vi "AutofocusContinuous.vi"() -> ()   [LabVIEW 2019]
uses:
  <vilib>/userDefined/High Color/IMAQdx.ctl
  include/GlobalVariables.vi
  Other Models/2010/Motion/AbortSingle.vi
  <vilib>/vision/NI_Vision_Development_Module.lvlib
  <vilib>/vision/driver/NI_Vision_Acquisition_Software.lvlib
panel:
  out "Array 2":sgl[][](array[numeric])
  out "Array":dbl[][](array[numeric])
  in  "StopAfterMaxFrac":dbl=0.7 format="%#_13g"
  out "Numeric Control 2":i32
  out "XY Graph":T1(graph)
  out "TimeTaken":dbl
  in  "Camera":T2="cam1"
  out "MaxVal":dbl
  out "BestZ":dbl
  out "SDvsZ":string
  out "Sobel_SD":picture
  in  "Z OutputFile":path=path "C:/Users/TTUHEP/Documents/LabVIEW/GantryPrograms/Configs/temp.txt"
  in  "Plot Output File":string="C:\\Users\\TTUHEP\\Documents\\LabVIEW\\GantryPrograms\\LogFiles\\plot.png"
  out "spreadsheet string":string
  out "Image":T3(plugin-control)
  in  "ScanRange":dbl=0.2
  out "error out":errorcluster
  in  "error in (no error)":errorcluster
  in  "Z":dbl=70.35
  in  "Y":dbl=982.4982903
  in  "X":dbl=291.0122844
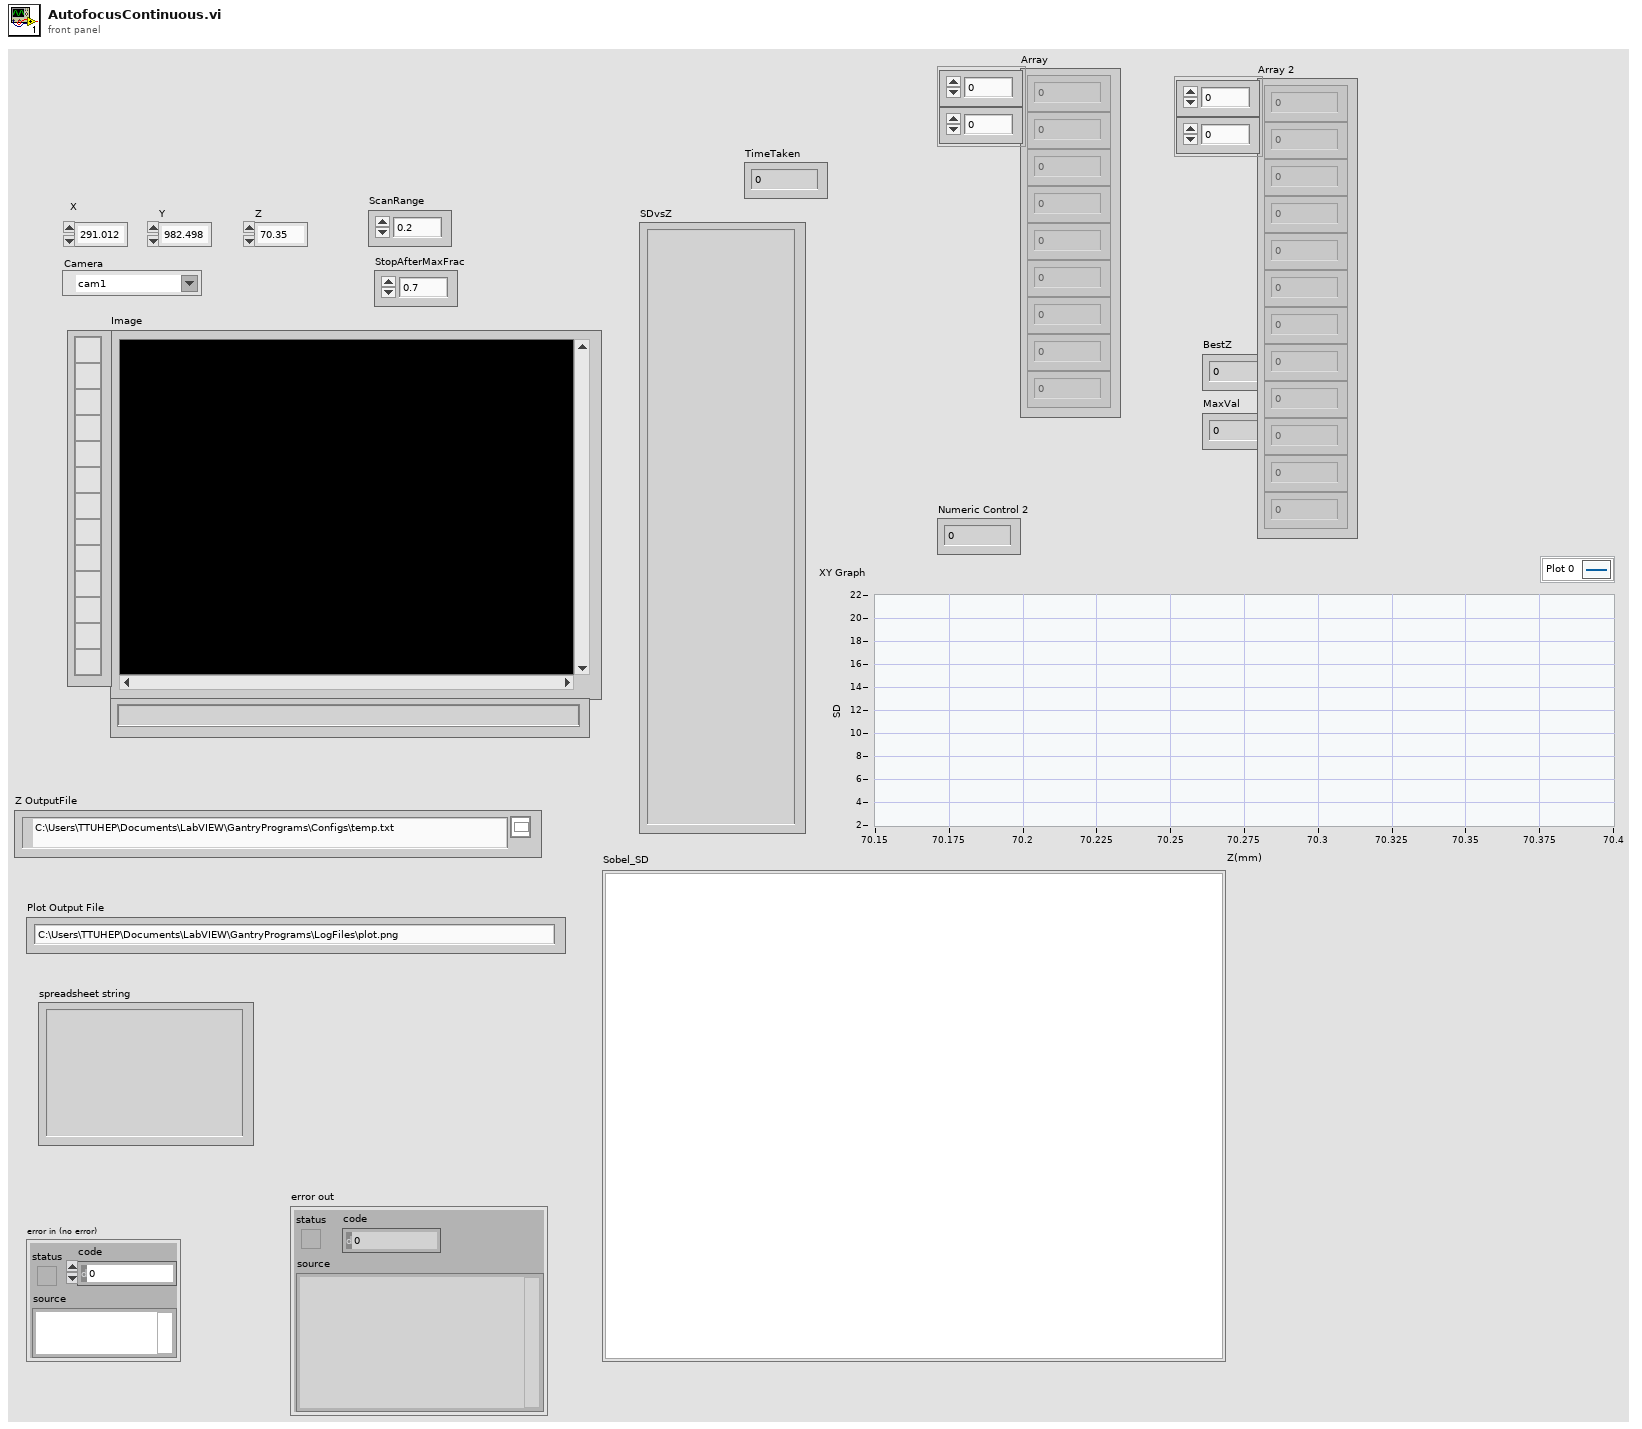
[diagram p1: front panel]
types:
  T1 = cluster{"Position Z":dbl, "Standard  Deviation":sgl}[]
  T2 = typedef "IMAQdx.ctl" = refnum<k21>
  T3 = typedef "IMAQ Image.ctl" = refnum<image>
  T4 = typedef "Image Type" = u32
  T5 = enum16{"open", "replace", "create", "open or create", "replace or create", "replace or create with confirmation"}
  T6 = enum32{"Differentiation", "Gradient", "Prewitt", "Roberts", "Sigma", "Sobel"}
  T7 = cluster{"Position Z":dbl, "Standard  Deviation":sgl}
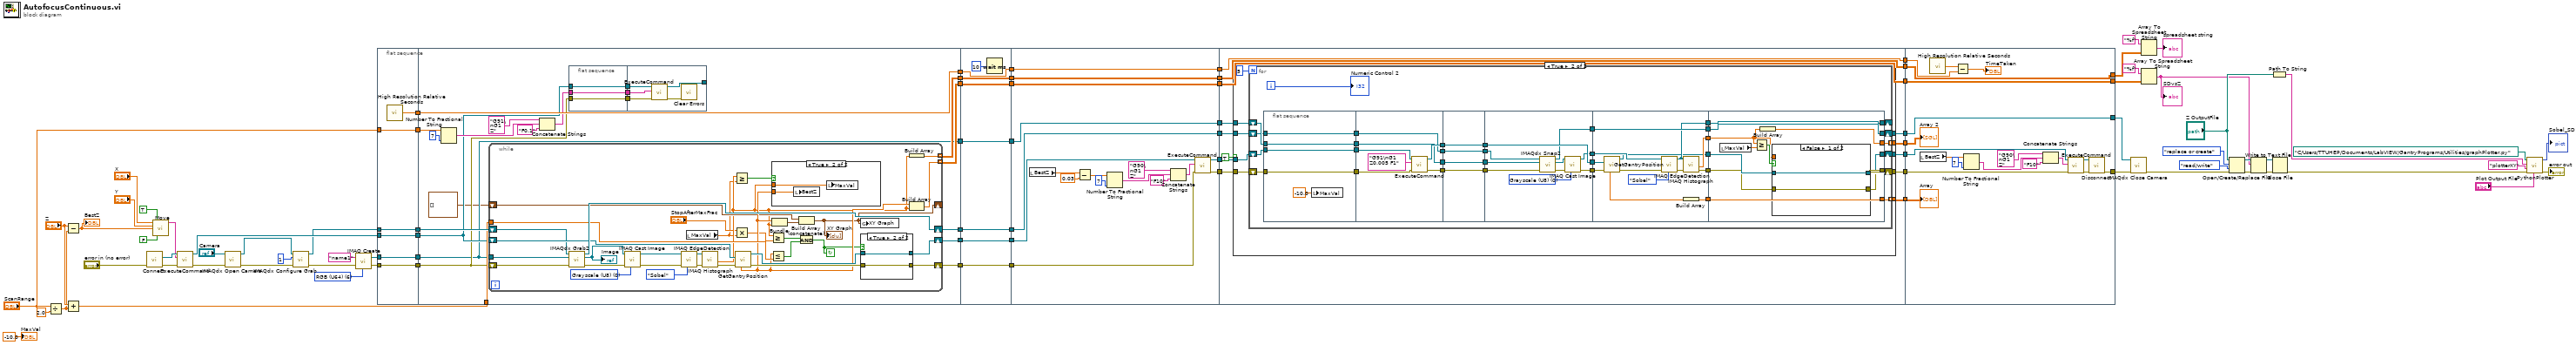
[diagram p0: block diagram]
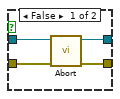
[diagram p2: hidden frame]
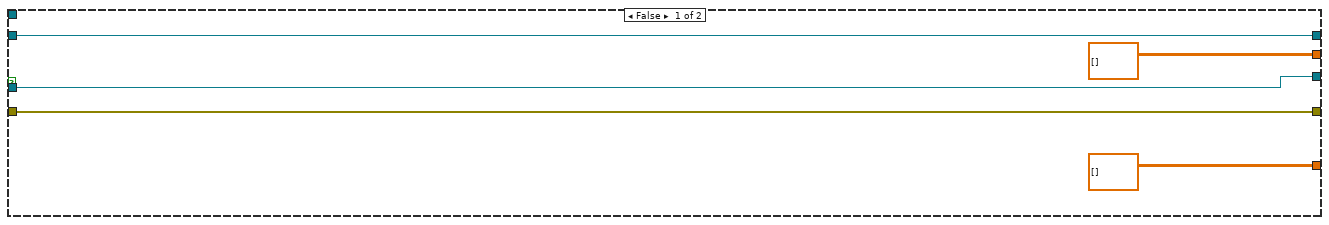
[diagram p4: hidden frame]
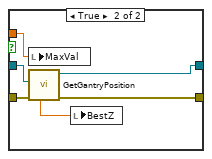
[diagram p5: hidden frame]
diagram:
  w53 = T4 6 items=["Grayscale (U8)", "Grayscale (I16)", "Grayscale (SGL)", "Complex (CSG)", "RGB (U32)", "HSL (U32)", "RGB (U64)", "Grayscale (U16)"] ("Image Type")
  n1 = Divide(x="ScanRange", y=2.0) -> (x/y=w34:dbl)
  n2 = Subtract(x="Z", y=w34) -> (x-y=w57:dbl)
  "BestZ" <- w57
  n3 = Add(x="Z", y=w34) -> (x+y=w33:dbl)
  n4 = call "Connect.vi"("error in (no error)"="error in (no error)") -> ("error out"=w48:errorcluster, "controller"=w79:refnum<k24>)  [unwired: 9 in]
  n5 = call "Move.vi"("X"="X", "Absolute"=TRUE, "Y"="Y", "Z"=w57, "Move Z first"=FALSE) -> ("Position Gcode"=w78:string)  [unwired: 10 in]
  n6 = call "ExecuteCommand.vi"("error in (no error)"=w48, "Command Code"=w78, "controller in"=w79) -> ("error out"=w47:errorcluster, "controller out"=w77:refnum<k24>)  [unwired: 6 in, 1 out]
  n7 = call <vilib>:"IMAQdx Open Camera.vi"("error in"=w47, "Session In"="Camera") -> ("error out"=w43:errorcluster, "Session Out"=w45:T2)  [unwired: 8 in]
  n8 = call <vilib>:"IMAQdx Configure Grab.vi"("error in"=w43, "Number of Buffers"=u32 1, "Session In"=w45) -> ("error out"=w42:errorcluster, "Session Out"=w44:T2)  [unwired: 7 in]
  n9 = call "IMAQ Create"("Image Name"="name1" ("ImageName"), "Image Type"=w53, "error in (no error)"=w42) -> ("New Image"=w52:T3, "error out"=w46:errorcluster)  [unwired: 2 in]
  n10 = flat-sequence {
    tunnel: w44 -> [w87]
    tunnel: w46 -> [w88]
    tunnel: w52 -> [w89]
    tunnel: "ScanRange" -> [w90]
    tunnel: w77 -> [w91]
    tunnel: [w91] -> w41
    tunnel: [w90] -> w40
    tunnel: [w89] -> w39
    tunnel: [w88] -> w38
    tunnel: [w87] -> w37
    tunnel: [w86] -> w36
    tunnel: w41 -> [w99]
    tunnel: w40 -> [w112]
    tunnel: w39 -> [w94]
    tunnel: w38 -> [w98]
    tunnel: w37 -> [w107]
    tunnel: [w93] -> w24
    tunnel: [w111] -> w22
    tunnel: [w110] -> w20
    tunnel: [w109] -> w18
    tunnel: [w108] -> w16
    tunnel: w36 -> [w106]
    tunnel: [w106] -> w14
    tunnel: w33 -> [w100]
    tunnel: [w94] -> w12
    tunnel: w24 -> [w169]
    tunnel: [w169] -> w23
    tunnel: w22 -> [w168]
    tunnel: [w168] -> w21
    tunnel: w20 -> [w167]
    tunnel: [w167] -> w19
    tunnel: w18 -> [w166]
    tunnel: [w166] -> w17
    tunnel: w16 -> [w165]
    tunnel: [w165] -> w15
    tunnel: w14 -> [w164]
    tunnel: [w164] -> w13
    tunnel: w12 -> [w163]
    tunnel: [w163] -> w11
    tunnel: w23 -> [w183]
    tunnel: w21 -> [w186]
    tunnel: w19 -> [w185]
    tunnel: w17 -> [w184]
    tunnel: w15 -> [w177]
    tunnel: w13 -> [w171]
    tunnel: [w186] -> w10
    tunnel: [w185] -> w9
    tunnel: [w184] -> w8
    tunnel: [w173] -> w7
    tunnel: w11 -> [w173]
    tunnel: [w172] -> w6
    tunnel: [w171] -> w5
    tunnel: [w170] -> w4
    tunnel: w10 -> [w199]
    tunnel: w9 -> [w198]
    tunnel: w8 -> [w197]
    tunnel: w7 -> [w195]
    tunnel: w6 -> [w193]
    tunnel: [w199] -> w31
    tunnel: [w198] -> w30
    tunnel: [w196] -> w29
    tunnel: [w194] -> w28
    tunnel: [w192] -> w27
    tunnel: w5 -> [w192]
    tunnel: [w190] -> w26
    tunnel: w4 -> [w191]
    tunnel: [w189] -> w3
    tunnel: [w188] -> w2
    tunnel: [w309] -> w50
    tunnel: [w322] -> w51
    tunnel: [w323] -> w60
    tunnel: [w324] -> w62
    tunnel: w31 -> [w324]
    tunnel: w30 -> [w323]
    tunnel: w29 -> [w322]
    tunnel: w28 -> [w310]
    tunnel: w27 -> [w320]
    tunnel: w26 -> [w313]
    tunnel: w3 -> [w307]
    tunnel: w2 -> [w306]
    frame #0 {
      n11 = call <vilib>:"High Resolution Relative Seconds.vi"() -> ("relative seconds"=w86:dbl)
    }
    frame #1 {
      n12 = Number To Fractional String(number=w112, precision (6)=i16 7) -> (F-format string=w103:string)  [unwired: 2 in]
      n13 = while {
        tunnel: [w145] -> w111 mode=indexing
        tunnel: [w144] -> w110 mode=indexing
        tunnel: w94 -> [w143]
        shift-right: [w142] -> w109
        shift-left: w107 -> [w113]
        shift-right: [w127] -> w93
        shift-left: w99 -> [w135]
        shift-right: [w125] -> w108
        shift-left: w98 -> [w131]
        tunnel: w100 -> [w129]
        shift-right: [w121] -> _
        shift-left: T1 [] -> [w122]
        stop <- w114 continue-if-true
        w139 = T4 0 items=["Grayscale (U8)", "Grayscale (I16)", "Grayscale (SGL)", "Complex (CSG)", "RGB (U32)", "HSL (U32)", "RGB (U64)", "Grayscale (U16)"] ("Image Type")
        n14 = call <vilib>:"IMAQdx Grab2.vi"("error in"=w131, "Image In"=w143, "Session In"=w113) -> ("error out"=w130:errorcluster, "Image Out"=w132:T3, "Session Out"=w142:T2)  [unwired: 5 in, 1 out]
        "Image" <- w132
        n15 = call "IMAQ Cast Image"("Image Type"=w139, "error in (no error)"=w130, "Image Src"=w132) -> ("error out"=w141:errorcluster, "Image Dst Out"=w140:T3)  [unwired: 7 in]
        n16 = call "IMAQ EdgeDetection"("Method"=T6."Sobel", "error in (no error)"=w141, "Image Src"=w140) -> ("error out"=w138:errorcluster, "Image Dst Out"=w137:T3)  [unwired: 7 in]
        n17 = local read "MaxVal"() -> (w118:dbl)
        n18 = call "IMAQ Histograph"("error in (no error)"=w138, "Image"=w137) -> ("error out"=w134:errorcluster, "Standard  Deviation"=w120:sgl)  [unwired: 6 in, 2 out]
        n19 = Greater Or Equal?(x=w120, y=w118) -> (x >= y?=w133:bool)
        n20 = Multiply(x="StopAfterMaxFrac", y=w118) -> (x*y=w117:dbl)
        n21 = call "GetGantryPosition.vi"("error in (no error)"=w134, "Controller In"=w135) -> ("error out"=w126:errorcluster, "controller out"=w128:refnum<k24>, "Position Z"=w124:dbl)  [unwired: 3 in, 4 out]
        n22 = Greater Or Equal?(x=w120, y=w117) -> (x >= y?=w116:bool)
        n23 = Less Or Equal?(x=w124, y=w129) -> (x <= y?=w115:bool)
        n24 = case shown="True" w133 {
          tunnel: w120 -> [_ w153]
          tunnel: w124 -> [_ w152]
          frame False {
          }
          frame True {
            n25 = local write "BestZ"(w152) -> ()
            n26 = local write "MaxVal"(w153) -> ()
          }
        }
        n27 = Bundle("Position Z"=w124, "Standard  Deviation"=w120) -> (w123:T7)  [unwired: 1 in]
        n28 = Build Array (concatenate)(w122, w123) -> (w121:T1)
        "XY Graph" <- w121
        n29 = And(x=w116, y=w115) -> (x .and. y?=w114:bool)
        n30 = global write "GlobalVariables.vi" "XY Graph"(w121) -> ()
        n31 = case shown="True" w114 {
          tunnel: w128 -> [w149 w151]
          tunnel: [w148 w151] -> w127
          tunnel: w126 -> [w147 w150]
          tunnel: [w146 w150] -> w125
          frame False {
            n32 = call-poly "Abort.vi"("error in (no error)"=w147, "controller in"=w149) -> ("error out"=w146:errorcluster, "controller out"=w148:refnum<k24>)  [unwired: 8 in]
          }
          frame True {
          }
        }
        n33 = Build Array(w120) -> (w145:sgl[])
        n34 = Build Array(w124, w120) -> (w144:dbl[])
      }
      n35 = Concatenate Strings("G91\nG1 Z", w103, "F0.1" ("string")) -> (w102:string)
      n36 = flat-sequence {
        tunnel: w98 -> [w154]
        tunnel: w102 -> [w155]
        tunnel: w99 -> [w156]
        tunnel: [w156] -> w97
        tunnel: [w155] -> w96
        tunnel: [w154] -> w95
        tunnel: w97 -> [w161]
        tunnel: w96 -> [w160]
        tunnel: w95 -> [w159]
        tunnel: [w158] -> _
        frame #0 {
        }
        frame #1 {
          n37 = call "ExecuteCommand.vi"("error in (no error)"=w159, "Command Code"=w160, "controller in"=w161) -> ("error out"=w157:errorcluster, "controller out"=w158:refnum<k24>)  [unwired: 6 in, 1 out]
          n38 = call <vilib>:"Clear Errors.vi"("error in (no error)"=w157) -> ()  [unwired: 5 in, 2 out]
        }
      }
    }
    frame #2 {
      n39 = Wait (ms)(milliseconds to wait=u32 10) -> ()  [unwired: 1 out]
    }
    frame #3 {
      n40 = local read "BestZ"() -> (w176:dbl)
      n41 = Subtract(x=w176, y=0.03) -> (x-y=w174:dbl)
      n42 = Number To Fractional String(number=w174, precision (6)=i16 7) -> (F-format string=w179:string)  [unwired: 2 in]
      n43 = Concatenate Strings("G90\nG1 Z", w179, "F10" ("string")) -> (w178:string)
      n44 = call "ExecuteCommand.vi"("error in (no error)"=w177, "Command Code"=w178, "controller in"=w183) -> ("error out"=w172:errorcluster, "controller out"=w170:refnum<k24>)  [unwired: 6 in, 1 out]
    }
    frame #4 {
      n45 = case shown="True" TRUE {
        tunnel: w197 -> [w200 w214]
        tunnel: [w200 w213] -> w196
        tunnel: w195 -> [_ w212]
        tunnel: [w203 w211] -> w194
        tunnel: w193 -> [w203 w210]
        tunnel: w191 -> [w204 w208]
        tunnel: [w204 w207] -> w190
        tunnel: [dbl[][] [] w206] -> w189
        tunnel: [sgl[][] [] w205] -> w188
        frame False {
        }
        frame True {
          n46 = for {
            N: 5 -> [_]
            shift-right: [w237] -> w213
            shift-left: w214 -> [w223]
            shift-right: [w238] -> w211
            shift-left: w210 -> [w247]
            shift-right: [w239] -> w207
            shift-left: w208 -> [w246]
            shift-right: [w225] -> _
            shift-left: w212 -> [w229]
            tunnel: [w221] -> w206 mode=indexing
            tunnel: [w220] -> w205 mode=indexing
            i -> [w234]
            n47 = flat-sequence {
              tunnel: w223 -> [w249]
              tunnel: w229 -> [w250]
              tunnel: w246 -> [w251]
              tunnel: w247 -> [w252]
              tunnel: [w252] -> w218
              tunnel: [w251] -> w217
              tunnel: [w250] -> w216
              tunnel: [w249] -> w215
              tunnel: [w258] -> w233
              tunnel: [w257] -> w231
              tunnel: [w254] -> w227
              tunnel: [w253] -> w224
              tunnel: w218 -> [w256]
              tunnel: w217 -> [w255]
              tunnel: w216 -> [w254]
              tunnel: w215 -> [w253]
              tunnel: w233 -> [w263]
              tunnel: [w263] -> w232
              tunnel: w231 -> [w262]
              tunnel: [w262] -> w230
              tunnel: [w261] -> w228
              tunnel: w227 -> [w261]
              tunnel: w224 -> [w260]
              tunnel: [w260] -> w222
              tunnel: w232 -> [w272]
              tunnel: w230 -> [w273]
              tunnel: [w273] -> w245
              tunnel: [w268] -> w244
              tunnel: [w267] -> w243
              tunnel: [w266] -> w235
              tunnel: w228 -> [w265]
              tunnel: w222 -> [w264]
              tunnel: w245 -> [w277]
              tunnel: w244 -> [w275]
              tunnel: w243 -> [w284]
              tunnel: [w276] -> w242
              tunnel: [w283] -> w241
              tunnel: [w282] -> w240
              tunnel: [w281] -> w236
              tunnel: w235 -> [w281]
              tunnel: [w280] -> w226
              tunnel: [w279] -> w219
              tunnel: w242 -> [w295]
              tunnel: w241 -> [w294]
              tunnel: w240 -> [w289]
              tunnel: [w293] -> w239
              tunnel: [w292] -> w238
              tunnel: [w291] -> w237
              tunnel: w236 -> [w291]
              tunnel: w226 -> [w290]
              tunnel: [w290] -> w225
              tunnel: [w288] -> w221
              tunnel: [w287] -> w220
              tunnel: w219 -> [w288]
              frame #0 {
                n48 = local write "MaxVal"(-10.0) -> ()
              }
              frame #1 {
                n49 = call "ExecuteCommand.vi"("error in (no error)"=w256, "Command Code"="G91\nG1 Z0.005 F1", "controller in"=w255) -> ("error out"=w258:errorcluster, "controller out"=w257:refnum<k24>)  [unwired: 6 in, 1 out]
              }
              frame #2 {
              }
              frame #3 {
                w271 = T4 0 items=["Grayscale (U8)", "Grayscale (I16)", "Grayscale (SGL)", "Complex (CSG)", "RGB (U32)", "HSL (U32)", "RGB (U64)", "Grayscale (U16)"] ("Image Type")
                n50 = call <vilib>:"IMAQdx Snap2.vi"("error in"=w272, "Image In"=w265, "Session In"=w264) -> ("error out"=w270:errorcluster, "Image Out"=w269:T3, "Session Out"=w266:T2)  [unwired: 6 in]
                n51 = call "IMAQ Cast Image"("Image Type"=w271, "error in (no error)"=w270, "Image Src"=w269) -> ("error out"=w268:errorcluster, "Image Dst Out"=w267:T3)  [unwired: 7 in]
              }
              frame #4 {
                n52 = call "GetGantryPosition.vi"("error in (no error)"=w275, "Controller In"=w277) -> ("error out"=w274:errorcluster, "controller out"=w276:refnum<k24>, "Position Z"=w278:dbl)  [unwired: 3 in, 4 out]
                n53 = call "IMAQ EdgeDetection"("Method"=T6."Sobel", "error in (no error)"=w274, "Image Src"=w284) -> ("error out"=w286:errorcluster, "Image Dst Out"=w280:T3)  [unwired: 7 in]
                n54 = call "IMAQ Histograph"("error in (no error)"=w286, "Image"=w280) -> ("error out"=w283:errorcluster, "Standard  Deviation"=w282:sgl)  [unwired: 6 in, 2 out]
                n55 = Build Array(w278) -> (w279:dbl[])
              }
              frame #5 {
                n56 = local read "MaxVal"() -> (w297:dbl)
                n57 = Greater Or Equal?(x=w289, y=w297) -> (x >= y?=w296:bool)
                n58 = Build Array(w289) -> (w287:sgl[])
                n59 = case shown="False" w296 {
                  tunnel: w289 -> [_ w300]
                  tunnel: w295 -> [w298 w305]
                  tunnel: [w298 w302] -> w293
                  tunnel: w294 -> [w299 w304]
                  tunnel: [w299 w303] -> w292
                  frame False {
                  }
                  frame True {
                    n60 = local write "MaxVal"(w300) -> ()
                    n61 = call "GetGantryPosition.vi"("error in (no error)"=w304, "Controller In"=w305) -> ("error out"=w303:errorcluster, "controller out"=w302:refnum<k24>, "Position Z"=w301:dbl)  [unwired: 3 in, 4 out]
                    n62 = local write "BestZ"(w301) -> ()
                  }
                }
              }
            }
            "Numeric Control 2" <- w234
          }
        }
      }
    }
    frame #5 {
      n63 = local read "BestZ"() -> (w308:dbl)
      n64 = call <vilib>:"High Resolution Relative Seconds.vi"() -> ("relative seconds"=w321:dbl)
      n65 = Subtract(x=w321, y=w320) -> (x-y=→"TimeTaken":dbl)
      n66 = Number To Fractional String(number=w308, precision (6)=i16 7) -> (F-format string=w315:string)  [unwired: 2 in]
      n67 = Concatenate Strings("G90\nG1 Z", w315, "F10" ("string")) -> (w314:string)
      n68 = call "ExecuteCommand.vi"("error in (no error)"=w310, "Command Code"=w314, "controller in"=w313) -> ("error out"=w312:errorcluster, "controller out"=w311:refnum<k24>)  [unwired: 6 in, 1 out]
      n69 = call "Disconnect.vi"("error in (no error)"=w312, "controller"=w311) -> ("error out"=w309:errorcluster)  [unwired: 9 in]
      "Array" <- w307
      "Array 2" <- w306
    }
  }
  n70 = call <vilib>:"IMAQdx Close Camera.vi"("error in"=w50, "Session In"=w51) -> ("error out"=w49:errorcluster)  [unwired: 9 in]
  n71 = Array To Spreadsheet String(array=w62, 3:"%f" ("format string")) -> (spreadsheet string=→"spreadsheet string":string)  [unwired: 1 in]
  n72 = Array To Spreadsheet String(array=w60, 3:"%f" ("format string")) -> (spreadsheet string=w58:string)  [unwired: 1 in]
  "SDvsZ" <- w58
  n73 = Open/Create/Replace File(file path (use dialog)="Z OutputFile", error in=w49, operation (0:open)=T5."replace or create", access (0:read/write)=enum16{"read/write", "read-only", "write-only"}."read/write") -> (refnum out=w70:refnum<file>, error out=w71:errorcluster)  [unwired: 2 in, 1 out]
  n74 = Write to Text File(file (use dialog)=w70, text=w58, error in=w71) -> (refnum out=w73:refnum<file>, error out=w72:errorcluster)  [unwired: 1 in, 1 out]
  n75 = Path To String(path="Z OutputFile") -> (string=w65:string)
  n76 = Close File(refnum=w73, error in=w72) -> (error out=w64:errorcluster)  [unwired: 1 out]
  n77 = call "PythonPlotter.vi"("Output File"="Plot Output File", "error in (no error)"=w64, "Function Name"="plotterXY", "Input File"=w65, "Python Path"=path "C:/Users/TTUHEP/Documents/LabVIEW/GantryPrograms/Utilities/graphPlotter.py") -> ("error out"=→"error out":errorcluster, "HighVSPosition"=→"Sobel_SD":picture)  [unwired: 4 in]
  "MaxVal" <- -10.0 ("MaxVal")
